vi "ParseRequest.vi"(10 "request variables Input":T1) -> (3 "DisplayRequest":string)   [LabVIEW 2011, in "Design Server.lvlib"]
uses:
  ADT 2/user project design.ctl
  AguaClara Design Server/Design Server.lvlib
panel:
  in  "file path (use dialog)":path
  out "request variables":cluster{"Key":string[], "Value":string[]}
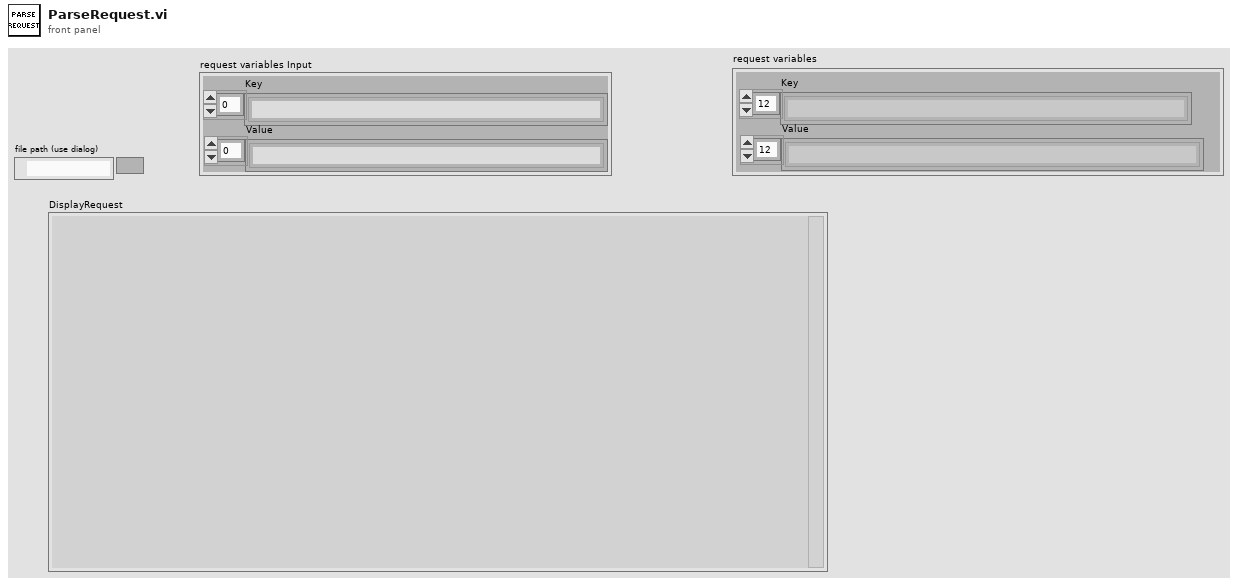
[diagram p1: front panel]
types:
  T1 = typedef "user project design.ctl" = cluster{"Key":string[], "Value":string[]}
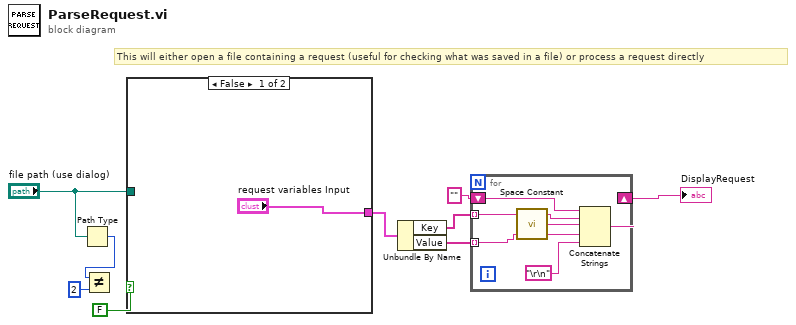
[diagram p0: block diagram]
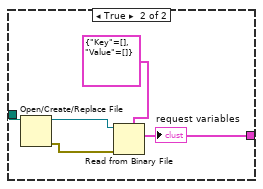
[diagram p2: hidden frame]
diagram:
  # "This will either open a file containing a request (useful for checking what was saved in a file) or process a request directly"
  n1 = Path Type(1:"file path (use dialog)") -> (0:w3:i16)
  n2 = Not Equal?(x=w3, y=i16 2 ("type")) -> ()  [unwired: 1 out]
  n3 = case shown="False" FALSE {
    tunnel: ["request variables Input" w12] -> w7
    tunnel: "file path (use dialog)" -> [_ w11]
    frame False {
    }
    frame True {
      n4 = Open/Create/Replace File(file path (use dialog)=w11) -> (refnum out=w14:refnum<file>, error out=w13:errorcluster)  [unwired: 5 in, 1 out]
      n5 = Read from Binary File(5:cluster{"Key":string[], "Value":string[]} {"Key"=[], "Value"=[]} ("request variables"), 8:w13, 11:w14) -> (2:w12:cluster{"Key":string[], "Value":string[]})  [unwired: 3 in, 3 out]
      "request variables" <- w12
    }
  }
  n6 = Unbundle By Name(w7) -> ("Key"=w6:string[], "Value"=w5:string[])
  n7 = for {
    shift-right: [w19] -> w8
    shift-left: "" -> [w20]
    tunnel: w6 -> [w18] mode=indexing
    tunnel: w5 -> [w17] mode=indexing
    n8 = call <vilib>:"Space Constant.vi"() -> ("String"=w16:string)
    n9 = Concatenate Strings(w20, w18, w16, w17, "\r\n") -> (w19:string)
  }
  "DisplayRequest" <- w8
